vi "global-body-transv.vi"(8 "Error In":errorcluster caption="错误输入", 10 "rad":dbl, 11 "Read?":bool=TRUE) -> (0 "Error Out":errorcluster caption="错误输入", 2 "rad out":dbl)   [LabVIEW 2013]
panel:
  # "本vi只记录角度, 转轴默认为y轴"
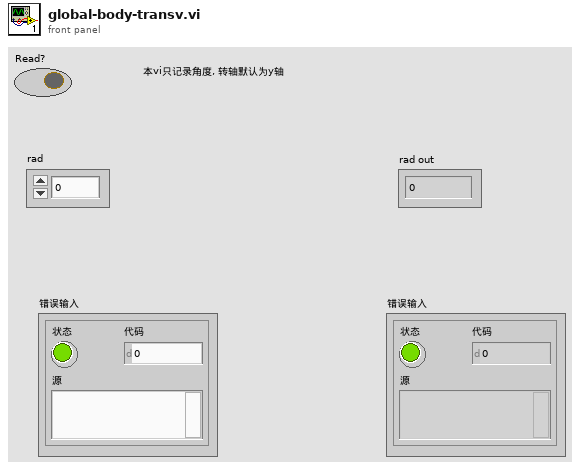
[diagram p1: front panel]
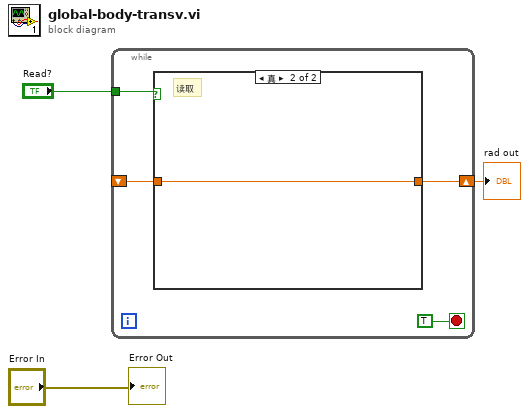
[diagram p0: block diagram]
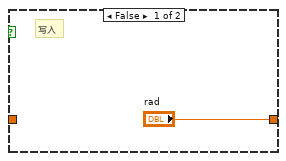
[diagram p2: hidden frame]
diagram:
  n1 = while {
    tunnel: "Read?" -> [w6]
    shift-right: [w5] -> w2
    shift-left: _ -> [w4]
    stop <- TRUE stop-if-true
    n2 = case shown="真" w6 {
      tunnel: ["rad" w9] -> w5
      tunnel: w4 -> [_ w9]
      frame False {
        # "写入"
      }
      frame True {
        # "读取"
      }
    }
  }
  "rad out" <- w2
  "Error Out" <- "Error In"
